vi "updateActuatorClosedLoop.vi"(8 "error in (no error)":errorcluster, 11 "Model in":refnum<class "Model.lvclass">) -> (0 "error out":errorcluster, 3 "Model out":refnum<class "Model.lvclass">)   [LabVIEW 2015, in "Model.lvclass"]
uses:
  Model.lvclass
  Typedefs/Actuate Settings.ctl
  Typedefs/ControlMode.ctl
  Model.lvclass/Model.ctl
  Actuator/IActuator/IActuator.lvclass
  Typedefs/FAMTTypedefs.lvlib
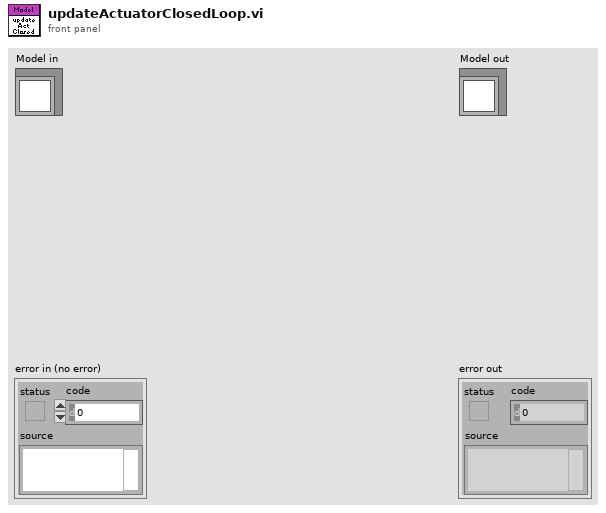
[diagram p1: front panel]
types:
  T1 = typedef "FAMTTypedefs.lvlib/Actuate Settings.ctl" = cluster{"Control Mode":T2, "Control Value":dbl, "Measured Value":dbl[unit], "FCV Value":dbl}
  T2 = typedef "FAMTTypedefs.lvlib/ControlMode.ctl" = enum16{"PSV", "FCV", "Both"}
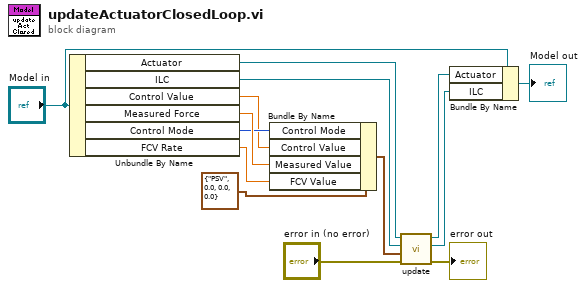
[diagram p0: block diagram]
diagram:
  n1 = Unbundle By Name("Model in") -> ("Actuator"=w14:refnum<class "IActuator.lvclass">, "ILC"=w10:refnum<class "ILC.lvclass">, "Control Value"=w1:dbl, "Measured Force"=w6:dbl[unit], "Control Mode"=w2:T2, "FCV Rate"=w5:dbl)
  n2 = Bundle By Name(cluster=T1 {"Control Mode"=enum."PSV", "Control Value"=0.0, "Measured Value"=0.0, "FCV Value"=0.0} ("Actuate Settings"), "Control Mode"=w2, "Control Value"=w1, "Measured Value"=w6, "FCV Value"=w5) -> (w7:T1)
  n3 = call-dynamic "update.vi"("error in (no error)"="error in (no error)", "Actuate Settings"=w7, "ILC in"=w10, "IActuator in"=w14) -> ("error out"=→"error out":errorcluster, "ILC out"=w9:refnum<class "ILC.lvclass">, "IActuator out"=w11:refnum<class "IActuator.lvclass">)  [unwired: 5 in]
  n4 = Bundle By Name(cluster="Model in", "Actuator"=w11, "ILC"=w9) -> (→"Model out":refnum<class "Model.lvclass">)
